vi "Recieve Data.vi"(8 "error in (no error)":errorcluster, 10 "Points to read":i32, 11 "RP Instrument in":refnum<class "RP Instrument.lvclass">) -> (0 "error out":errorcluster, 2 "Data out":i32[](array[numeric]), 3 "RP Instrument out":refnum<class "RP Instrument.lvclass">)   [LabVIEW 2015, in "RP Instrument.lvclass"]
uses:
  RP Instrument.lvclass
  RP Instrument.lvclass/RP Instrument.ctl
  RP Communicator/RP Communicator.lvclass
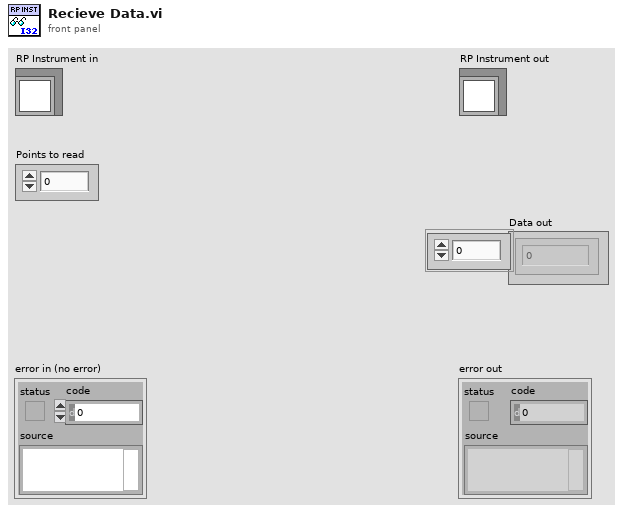
[diagram p1: front panel]
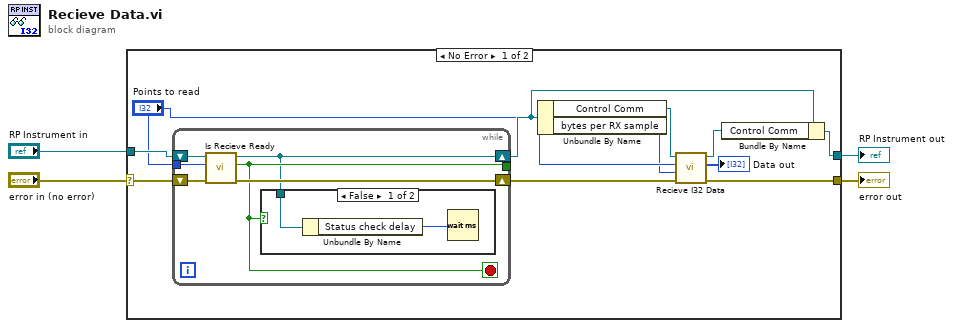
[diagram p0: block diagram]
diagram:
  n1 = case shown="No Error" "error in (no error)" {
    selector: "error in (no error)" -> [w10 w25]
    tunnel: [w11 w25] -> w3
    tunnel: [w12 w24] -> w1
    tunnel: "RP Instrument in" -> [w7 w24]
    frame No Error {
      n2 = while {
        shift-right: [w19] -> w9
        shift-left: w10 -> [w20]
        shift-right: [w16] -> w8
        shift-left: w7 -> [w21]
        tunnel: [w18] -> _
        tunnel: "Points to read" -> [w17]
        stop <- w18 stop-if-true
        n3 = call-dynamic "Is Recieve Ready.vi"("error in (no error)"=w20, "Points to read"=w17, "RP Instrument in"=w21) -> ("error out"=w19:errorcluster, "Recieve Ready"=w18:bool, "RP Instrument out"=w16:refnum<class "RP Instrument.lvclass">)  [unwired: 5 in, 1 out]
        n4 = case shown="False" w18 {
          tunnel: w16 -> [w23 _]
          frame False {
            n5 = Unbundle By Name(w23) -> ("Status check delay"=w22:u32)
            n6 = Wait (ms)(milliseconds to wait=w22) -> ()  [unwired: 1 out]
          }
          frame True {
          }
        }
      }
      n7 = Unbundle By Name(w8) -> ("Control Comm"=w13:refnum<class "RP Communicator.lvclass">, "bytes per RX sample"=w5:u32)
      n8 = call-dynamic "Recieve I32 Data.vi"("error in (no error)"=w9, "bytes per sample"=w5, "Samples per read"="Points to read", "RP Communicator in"=w13) -> ("error out"=w11:errorcluster, "Data out"=→"Data out":i32[], "RP Communicator out"=w14:refnum<class "RP Communicator.lvclass">)  [unwired: 5 in]
      n9 = Bundle By Name(cluster=w8, "Control Comm"=w14) -> (w12:refnum<class "RP Instrument.lvclass">)
    }
    frame Error {
    }
  }
  "error out" <- w3
  "RP Instrument out" <- w1
